vi "DialogLoop.vi"(8 "Error In":errorcluster, 11 "Message Queues":T1) -> (0 "Error Out":errorcluster)   [LabVIEW 2017, in "Server.lvlib" / "Dialogs.lvlib"]
doc: "This Loop can launch several Dialogs as asyncronous Popup-VIs."
uses:
  Dialogs.lvlib
  Message Queue/CommReferences.ctl
  Message Queue/MessageCluster.ctl
  DialogLoopData.ctl
  TypeDefs/ServerINI.ctl
  Oracle/OracleData.ctl
  TypeDefs/ClientConfiguration.ctl
  <vilib>/Utility/error.llb/Error Cluster From Error Code.vi
  <vilib>/ErrorRing/Error Ring.xnode
  Message Queue/Message Queue.lvlib
  ErrorLogger/ErrorLogger.lvlib
  Oracle/Oracle.lvlib
  Server.lvlib
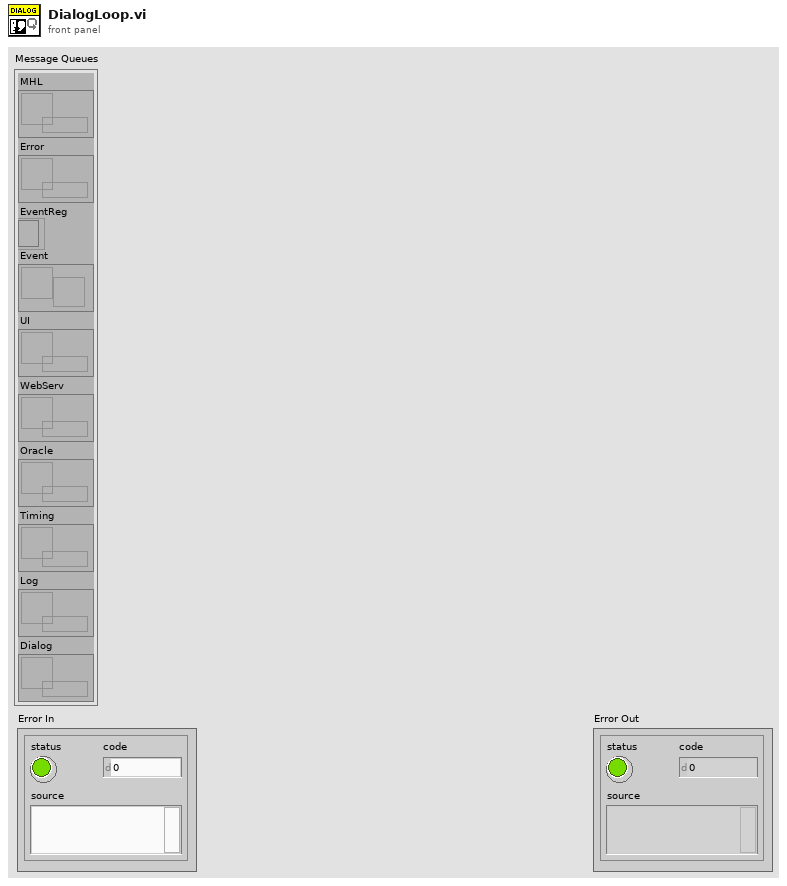
[diagram p1: front panel]
types:
  T1 = typedef "Server.lvlib/Message Queue.lvlib/CommReferences.ctl" = cluster{"MHL":refnum<queue>, "Error":refnum<queue>, "EventReg":refnum<event-registration>, "Event":refnum<user-event>, "UI":refnum<queue>, "WebServ":refnum<queue>, "Oracle":refnum<queue>, "Timing":refnum<queue>, "Log":refnum<queue>, "Dialog":refnum<queue>}
  T2 = typedef "Server.lvlib/Dialogs.lvlib/DialogLoopData.ctl" = cluster{"ServerINI":T3}
  T3 = typedef "Server.lvlib/ServerINI.ctl" = cluster{"ClientTimeout (s)":u32, "LogPath":path, "ErrorsToIgnore":i32[], "OracleData":T4, "ClientConfig":T5}
  T4 = typedef "Server.lvlib/Oracle.lvlib/OracleData.ctl" = cluster{"DBname":string, "User":string, "Password":string}
  T5 = typedef "Server.lvlib/ClientConfiguration.ctl" = cluster{"ColorCodes":u32[]}
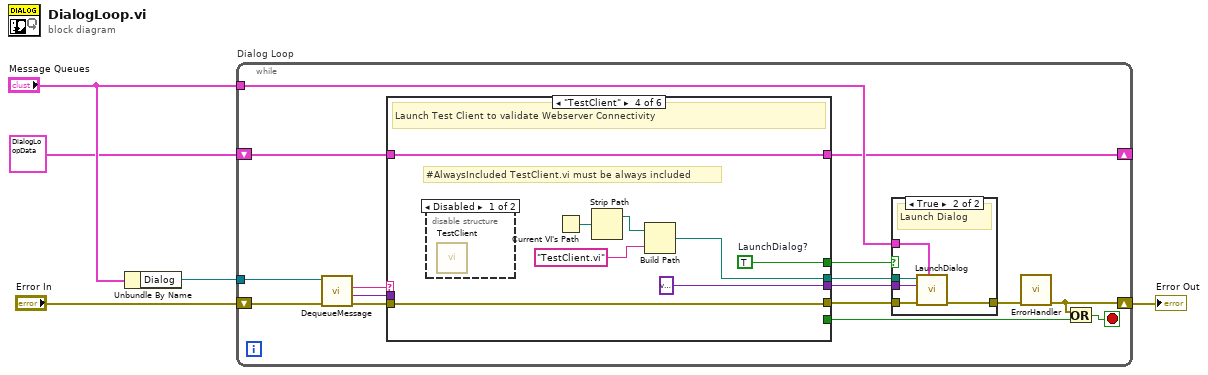
[diagram p0: block diagram]
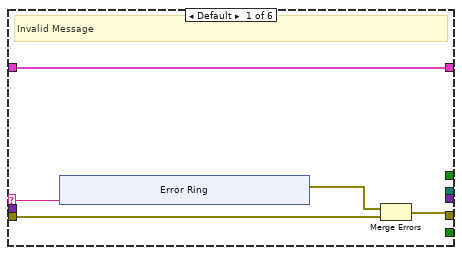
[diagram p3: hidden frame]
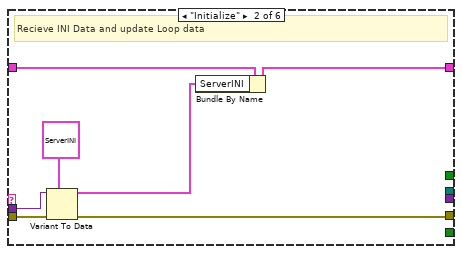
[diagram p4: hidden frame]
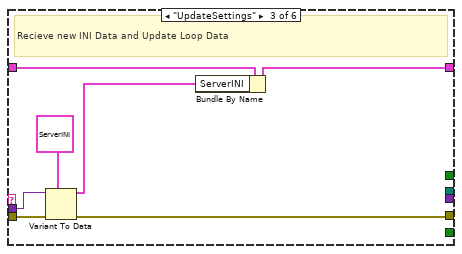
[diagram p5: hidden frame]
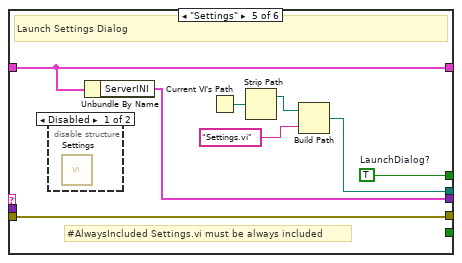
[diagram p7: hidden frame]
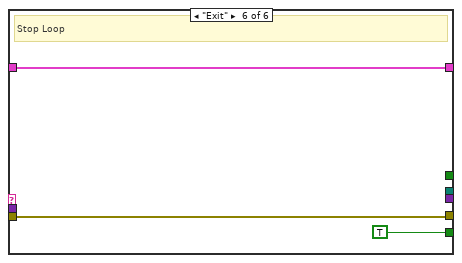
[diagram p9: hidden frame]
diagram:
  n1 = Unbundle By Name("Message Queues") -> ("Dialog"=w5:refnum<queue>)
  n2 = while "Dialog Loop" {
    shift-right: [w6] -> w4
    shift-left: "Error In" -> [w21]
    tunnel: w5 -> [w20]
    tunnel: "Message Queues" -> [w11]
    shift-right: [w8] -> _
    shift-left: T2 {"ServerINI"={"ClientTimeout (s)"=30, "LogPath"=path "C:/Users/jgoebel/Documents/GitHub/AEDashboard/ServerLib/Data/ServerLog.tdms", "ErrorsToIgnore"=[], "OracleData"={"DBname"="", "User"="", "Password"=""}, "ClientConfig"={"ColorCodes"=[16711680, 6618880, 16774745, 9567230]}}} ("DialogLoopData") -> [w9]
    stop <- w7 stop-if-true
    n3 = call "DequeueMessage.vi"("error in (no error)"=w21, "Message Queue"=w20) -> ("error out"=w19:errorcluster, "Message Data"=w17:variant, "Message"=w15:string)  [unwired: 5 in, 2 out]
    n4 = case shown="\"TestClient\"" w15 {
      selector: w15 -> [w31 _ _ _ _ _]
      tunnel: [w30 w45 w50 w61 w69 w72] -> w18
      tunnel: w19 -> [w32 w46 w53 w61 w69 w72]
      tunnel: w17 -> [_ w44 w49 _ _ _]
      tunnel: [_ _ _ _ _ TRUE] -> w16
      tunnel: [_ _ _ w55 w64 _] -> w13
      tunnel: [_ _ _ w60 w68 _] -> w12
      tunnel: [_ _ _ variant w62 _] -> w10
      tunnel: [w28 w41 w51 w54 w63 w70] -> w8
      tunnel: w9 -> [w28 w42 w52 w54 w63 w70]
      frame Default {
        # "Invalid Message"
        n5 = xnode "Error Ring"("parameter 0"=w31) -> ("error out"=w29:errorcluster)
        n6 = Merge Errors(w29, w32) -> (w30:errorcluster)
      }
      frame "Initialize" {
        # "Recieve INI Data and update Loop data"
        n7 = Variant To Data(error in=w46, type=T3 {"ClientTimeout (s)"=30, "LogPath"=path "C:/Users/jgoebel/Documents/GitHub/AEDashboard/ServerLib/Data/ServerLog.tdms", "ErrorsToIgnore"=[], "OracleData"={"DBname"="", "User"="", "Password"=""}, "ClientConfig"={"ColorCodes"=[16711680, 6618880, 16774745, 9567230]}} ("ServerINI"), Variant=w44) -> (data=w40:T3, error out=w45:errorcluster)
        n8 = Bundle By Name(cluster=w42, "ServerINI"=w40) -> (w41:T2)
      }
      frame "UpdateSettings" {
        # "Recieve new INI Data and Update Loop Data"
        n9 = Variant To Data(error in=w53, type=T3 {"ClientTimeout (s)"=30, "LogPath"=path "C:/Users/jgoebel/Documents/GitHub/AEDashboard/ServerLib/Data/ServerLog.tdms", "ErrorsToIgnore"=[], "OracleData"={"DBname"="", "User"="", "Password"=""}, "ClientConfig"={"ColorCodes"=[16711680, 6618880, 16774745, 9567230]}} ("ServerINI"), Variant=w49) -> (data=w47:T3, error out=w50:errorcluster)
        n10 = Bundle By Name(cluster=w52, "ServerINI"=w47) -> (w51:T2)
      }
      frame "TestClient" {
        w60 = TRUE  # LaunchDialog?
        # "#AlwaysIncluded TestClient.vi must be always included"
        # "Launch Test Client to validate Webserver Connectivity"
        n11 = disable-structure shown="Disabled" {
          frame Disabled {
            n12 = call "TestClient.vi"() -> ()  [unwired: 12 in]
          }
          frame Enabled {
          }
        }
        n13 = Current VI's Path() -> (path=w58:path)
        n14 = Strip Path(path=w58) -> (stripped path=w57:path)  [unwired: 1 out]
        n15 = Build Path(base path=w57, name or relative path="TestClient.vi") -> (appended path=w55:path)
      }
      frame "Settings" {
        w68 = TRUE  # LaunchDialog?
        # "#AlwaysIncluded Settings.vi must be always included"
        # "Launch Settings Dialog"
        n16 = disable-structure shown="Disabled" {
          frame Disabled {
            n17 = call "Settings.vi"() -> ()  [unwired: 12 in]
          }
          frame Enabled {
          }
        }
        n18 = Unbundle By Name(w63) -> ("ServerINI"=w62:T3)
        n19 = Current VI's Path() -> (path=w67:path)
        n20 = Strip Path(path=w67) -> (stripped path=w66:path)  [unwired: 1 out]
        n21 = Build Path(base path=w66, name or relative path="Settings.vi") -> (appended path=w64:path)
      }
      frame "Exit" {
        # "Stop Loop"
      }
    }
    n22 = case shown="True" w12 {
      tunnel: w18 -> [w22 w27]
      tunnel: [w22 w26] -> w14
      tunnel: w13 -> [_ w25]
      tunnel: w11 -> [_ w24]
      tunnel: w10 -> [_ w23]
      frame False {
      }
      frame True {
        # "Launch Dialog"
        n23 = call "LaunchDialog.vi"("Queues"=w24, "error in (no error)"=w27, "DialogData"=w23, "DialogPath"=w25) -> ("error out"=w26:errorcluster)  [unwired: 7 in]
      }
    }
    n24 = call "ErrorHandler.vi"("error in (no error)"=w14) -> ("error out"=w6:errorcluster)  [unwired: 10 in]
    n25 = Or(x=w6, y=w16) -> (x .or. y?=w7:bool)
  }
  "Error Out" <- w4
